vi "check hit on image.vi"(8 "Cluster":cluster{"Numeric":i32, "Numeric 2":i32}, 10 "Array":cluster{"Numeric":i32, "Numeric 2":i32}[](array[cluster])) -> (1 "Array 2":cluster{"Numeric":i32, "Numeric 2":i32}[](array[cluster]), 3 "last target":bool)   [LabVIEW 2014]
panel:
  out "last target 2":bool
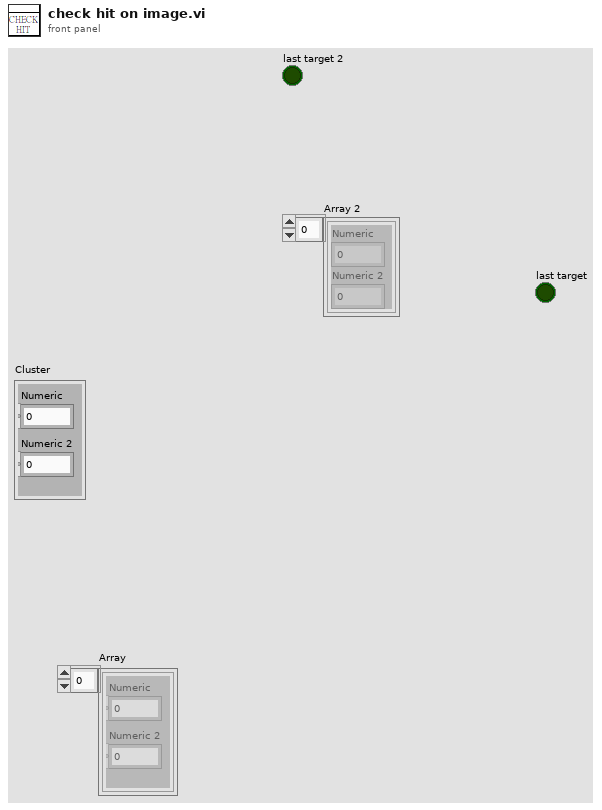
[diagram p1: front panel]
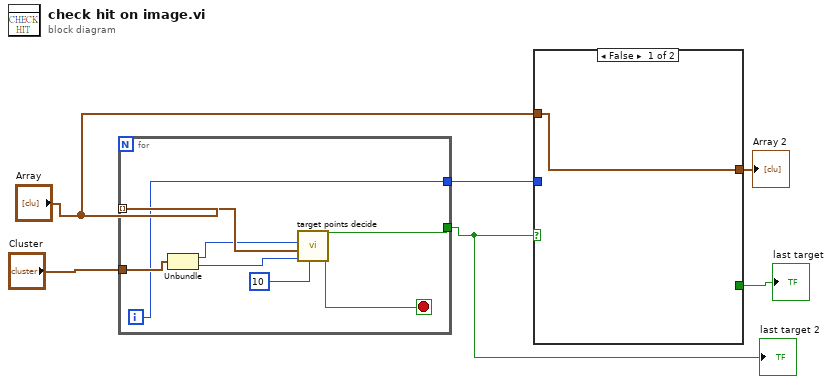
[diagram p0: block diagram]
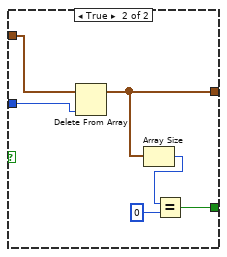
[diagram p2: hidden frame]
diagram:
  n1 = for {
    tunnel: "Array" -> [w12] mode=indexing
    tunnel: "Cluster" -> [w13]
    tunnel: [w9] -> w1
    tunnel: [w8] -> w4
    i -> [w8]
    stop <- w9 stop-if-true
    n2 = Unbundle(w13) -> ("Numeric"=w11:i32, "Numeric 2"=w10:i32)
    n3 = call "target points decide.vi"("Spacing limit"=10, "Y"=w10, "Cluster"=w12, "X"=w11) -> ("too close?"=w9:bool)  [unwired: 7 in]
  }
  "last target 2" <- w1
  n4 = case shown="False" w1 {
    tunnel: "Array" -> [w14 w20]
    tunnel: w4 -> [_ w19]
    tunnel: [w14 w18] -> w3
    tunnel: [_ w15] -> w2
    frame False {
    }
    frame True {
      n5 = Delete From Array(array=w20, index=w19) -> (array with subset deleted=w18:cluster{"Numeric":i32, "Numeric 2":i32}[])  [unwired: 1 in, 1 out]
      n6 = Array Size(array=w18) -> (size(s)=w17:i32)
      n7 = Equal?(x=w17, y=0) -> (x = y?=w15:bool)
    }
  }
  "Array 2" <- w3
  "last target" <- w2
